vi "input_channel_task.vi"(8 "error in":errorcluster, 10 "Analog Input Channels":T2[](array[typedef])=[{"Channel Name"="Vapor Mass Flow", "Physical Channel"="cDAQ1Mod2/ai5", "Sensor Type"=enum."Mass Flow Rate", "Signal Type"=enum."Current", "Terminal Configuration"=-1, "Minimum Value"=0.004, "Maximum Value"=0.02, "TC Type"=10086, "Sensor Min"=0.0, "Sensor Max"=50.0, "Sensor Offset"=0.0, "Sensor Unit"=enum."g/s", "Output Unit"=enum."g/s", "Unit Conversion"=1.0, "Active"=TRUE}, {"Channel Name"="Vapor Line Density", "Physical Channel"="cDAQ1Mod2/ai6", "Sensor Type"=enum."Density", "Signal Type"=enum."Current", "Terminal Configuration"=-1, "Minimum Value"=0.004, "Maximum Value"=0.02, "TC Type"=10086, "Sensor Min"=0.0, "Sensor Max"=50.0, "Sensor Offset"=0.0, "Sensor Unit"=enum."g/cm3", "Output Unit"=enum."g/cm3", "Unit Conversion"=1.0, "Active"=TRUE}, {"Channel Name"="Liquid Mass Flow", "Physical Channel"="cDAQ1Mod2/ai3", "Sensor Type"=enum."Mass Flow Rate", "Signal Type"=enum."Current", "Terminal Configuration"=-1, "Minimum Value"=0.004, "Maximum Value"=0.02, "TC Type"=10086, "Sensor Min"=0.0, "Sensor Max"=50.0, "Sensor Offset"=0.0, "Sensor Unit"=enum."g/s", "Output Unit"=enum."g/s", "Unit Conversion"=1.0, "Active"=TRUE}, {"Channel Name"="Liquid Line Density", "Physical Channel"="cDAQ1Mod2/ai4", "Sensor Type"=enum."Density", "Signal Type"=enum."Current", "Terminal Configuration"=-1, "Minimum Value"=0.004, "Maximum Value"=0.02, "TC Type"=10086, "Sensor Min"=0.0, "Sensor Max"=50.0, "Sensor Offset"=0.0, "Sensor Unit"=enum."g/cm3", "Output Unit"=enum."g/cm3", "Unit Conversion"=1.0, "Active"=TRUE}, {"Channel Name"="Vapor Tank Pressure", "Physical Channel"="cDAQ1Mod5/ai1", "Sensor Type"=enum."Absolute Pressure", "Signal Type"=enum."Voltage", "Terminal Configuration"=-1, "Minimum Value"=0.0, "Maximum Value"=5.0, "TC Type"=10086, "Sensor Min"=0.0, "Sensor Max"=50.0, "Sensor Offset"=0.0, "Sensor Unit"=enum."psi", "Output Unit"=enum."Pa", "Unit Conversion"=6894.75729, "Active"=TRUE}, {"Channel Name"="Liquid Tank Pressure", "Physical Channel"="cDAQ1Mod5/ai2", "Sensor Type"=enum."Absolute Pressure", "Signal Type"=enum."Voltage", "Terminal Configuration"=-1, "Minimum Value"=0.0, "Maximum Value"=5.0, "TC Type"=10086, "Sensor Min"=0.0, "Sensor Max"=50.0, "Sensor Offset"=0.0, "Sensor Unit"=enum."psi", "Output Unit"=enum."Pa", "Unit Conversion"=6894.75729, "Active"=TRUE}, {"Channel Name"="Separator Pressure", "Physical Channel"="cDAQ1Mod5/ai0", "Sensor Type"=enum."Absolute Pressure", "Signal Type"=enum."Voltage", "Terminal Configuration"=-1, "Minimum Value"=0.0, "Maximum Value"=5.0, "TC Type"=10086, "Sensor Min"=0.0, "Sensor Max"=50.0, "Sensor Offset"=0.0, "Sensor Unit"=enum."psi", "Output Unit"=enum."Pa", "Unit Conversion"=6894.75729, "Active"=TRUE}, {"Channel Name"="Liquid Inlet Pressure", "Physical Channel"="cDAQ1Mod5/ai4", "Sensor Type"=enum."Absolute Pressure", "Signal Type"=enum."Voltage", "Terminal Configuration"=-1, "Minimum Value"=0.0, "Maximum Value"=5.0, "TC Type"=10086, "Sensor Min"=0.0, "Sensor Max"=50.0, "Sensor Offset"=0.0, "Sensor Unit"=enum."psi", "Output Unit"=enum."Pa", "Unit Conversion"=6894.75729, "Active"=TRUE}, {"Channel Name"="Vapor Inlet Pressure", "Physical Channel"="cDAQ1Mod5/ai3", "Sensor Type"=enum."Absolute Pressure", "Signal Type"=enum."Voltage", "Terminal Configuration"=-1, "Minimum Value"=0.0, "Maximum Value"=5.0, "TC Type"=10086, "Sensor Min"=0.0, "Sensor Max"=50.0, "Sensor Offset"=0.0, "Sensor Unit"=enum."psi", "Output Unit"=enum."Pa", "Unit Conversion"=6894.75729, "Active"=TRUE}, {"Channel Name"="Vapor Tank Temperature", "Physical Channel"="cDAQ1Mod6/ai1", "Sensor Type"=enum."Temperature", "Signal Type"=enum."Temperature", "Terminal Configuration"=-1, "Minimum Value"=0.0, "Maximum Value"=100.0, "TC Type"=10086, "Sensor Min"=0.0, "Sensor Max"=50.0, "Sensor Offset"=0.0, "Sensor Unit"=enum."C", "Output Unit"=enum."C", "Unit Conversion"=1.0, "Active"=TRUE}, {"Channel Name"="Vapor Inlet Temperature", "Physical Channel"="cDAQ1Mod7/ai2", "Sensor Type"=enum."Temperature", "Signal Type"=enum."Temperature", "Terminal Configuration"=-1, "Minimum Value"=0.0, "Maximum Value"=100.0, "TC Type"=10086, "Sensor Min"=0.0, "Sensor Max"=50.0, "Sensor Offset"=0.0, "Sensor Unit"=enum."C", "Output Unit"=enum."C", "Unit Conversion"=1.0, "Active"=TRUE}, {"Channel Name"="Liquid Tank Temperature", "Physical Channel"="cDAQ1Mod6/ai2", "Sensor Type"=enum."Temperature", "Signal Type"=enum."Temperature", "Terminal Configuration"=-1, "Minimum Value"=0.0, "Maximum Value"=100.0, "TC Type"=10086, "Sensor Min"=0.0, "Sensor Max"=50.0, "Sensor Offset"=0.0, "Sensor Unit"=enum."C", "Output Unit"=enum."C", "Unit Conversion"=1.0, "Active"=TRUE}, {"Channel Name"="Liquid Inlet Temperature", "Physical Channel"="cDAQ1Mod7/ai3", "Sensor Type"=enum."Temperature", "Signal Type"=enum."Temperature", "Terminal Configuration"=-1, "Minimum Value"=0.0, "Maximum Value"=100.0, "TC Type"=10086, "Sensor Min"=0.0, "Sensor Max"=50.0, "Sensor Offset"=0.0, "Sensor Unit"=enum."C", "Output Unit"=enum."C", "Unit Conversion"=1.0, "Active"=TRUE}, {"Channel Name"="Separator Temperature", "Physical Channel"="cDAQ1Mod6/ai0", "Sensor Type"=enum."Temperature", "Signal Type"=enum."Temperature", "Terminal Configuration"=-1, "Minimum Value"=0.0, "Maximum Value"=100.0, "TC Type"=10086, "Sensor Min"=0.0, "Sensor Max"=50.0, "Sensor Offset"=0.0, "Sensor Unit"=enum."C", "Output Unit"=enum."C", "Unit Conversion"=1.0, "Active"=TRUE}, {"Channel Name"="Lower Dev Section Pressure", "Physical Channel"="cDAQ1Mod5/ai6", "Sensor Type"=enum."Absolute Pressure", "Signal Type"=enum."Voltage", "Terminal Configuration"=-1, "Minimum Value"=0.0, "Maximum Value"=5.0, "TC Type"=10086, "Sensor Min"=0.0, "Sensor Max"=50.0, "Sensor Offset"=0.0, "Sensor Unit"=enum."psi", "Output Unit"=enum."Pa", "Unit Conversion"=6894.75729, "Active"=TRUE}, {"Channel Name"="Upper Dev Section Temperature", "Physical Channel"="cDAQ1Mod6/ai3", "Sensor Type"=enum."Temperature", "Signal Type"=enum."Temperature", "Terminal Configuration"=-1, "Minimum Value"=0.0, "Maximum Value"=100.0, "TC Type"=10086, "Sensor Min"=0.0, "Sensor Max"=50.0, "Sensor Offset"=0.0, "Sensor Unit"=enum."C", "Output Unit"=enum."C", "Unit Conversion"=1.0, "Active"=TRUE}, {"Channel Name"="Upper Dev Section Pressure", "Physical Channel"="cDAQ1Mod5/ai5", "Sensor Type"=enum."Absolute Pressure", "Signal Type"=enum."Voltage", "Terminal Configuration"=-1, "Minimum Value"=0.0, "Maximum Value"=5.0, "TC Type"=10086, "Sensor Min"=0.0, "Sensor Max"=50.0, "Sensor Offset"=0.0, "Sensor Unit"=enum."psi", "Output Unit"=enum."Pa", "Unit Conversion"=6894.75729, "Active"=TRUE}, {"Channel Name"="Test Section Temperature", "Physical Channel"="cDAQ1Mod6/ai10", "Sensor Type"=enum."Temperature", "Signal Type"=enum."Temperature", "Terminal Configuration"=-1, "Minimum Value"=0.0, "Maximum Value"=100.0, "TC Type"=10086, "Sensor Min"=0.0, "Sensor Max"=50.0, "Sensor Offset"=0.0, "Sensor Unit"=enum."C", "Output Unit"=enum."C", "Unit Conversion"=1.0, "Active"=TRUE}, {"Channel Name"="Mixing Tee dP", "Physical Channel"="cDAQ1Mod5/ai9", "Sensor Type"=enum."Differential Pressure", "Signal Type"=enum."Voltage", "Terminal Configuration"=-1, "Minimum Value"=0.05, "Maximum Value"=5.05, "TC Type"=10086, "Sensor Min"=0.0, "Sensor Max"=50.0, "Sensor Offset"=0.0, "Sensor Unit"=enum."psi", "Output Unit"=enum."Pa", "Unit Conversion"=6894.75729, "Active"=TRUE}, {"Channel Name"="PG inlet-Mixing Tee Pressure", "Physical Channel"="cDAQ1Mod5/ai10", "Sensor Type"=enum."Absolute Pressure", "Signal Type"=enum."Voltage", "Terminal Configuration"=-1, "Minimum Value"=0.0, "Maximum Value"=5.0, "TC Type"=10086, "Sensor Min"=0.0, "Sensor Max"=50.0, "Sensor Offset"=0.0, "Sensor Unit"=enum."psi", "Output Unit"=enum."Pa", "Unit Conversion"=6894.75729, "Active"=TRUE}, {"Channel Name"="PG inlet-Mixing Tee Temperature", "Physical Channel"="cDAQ1Mod7/ai6", "Sensor Type"=enum."Temperature", "Signal Type"=enum."Temperature", "Terminal Configuration"=-1, "Minimum Value"=0.0, "Maximum Value"=100.0, "TC Type"=10073, "Sensor Min"=0.0, "Sensor Max"=50.0, "Sensor Offset"=0.0, "Sensor Unit"=enum."C", "Output Unit"=enum."C", "Unit Conversion"=1.0, "Active"=TRUE}, {"Channel Name"="Atmospheric Pressure", "Physical Channel"="cDAQ1Mod5/ai8", "Sensor Type"=enum."Absolute Pressure", "Signal Type"=enum."Voltage", "Terminal Configuration"=-1, "Minimum Value"=1.0, "Maximum Value"=5.0, "TC Type"=10086, "Sensor Min"=0.0, "Sensor Max"=50.0, "Sensor Offset"=0.0, "Sensor Unit"=enum."psi", "Output Unit"=enum."Pa", "Unit Conversion"=6894.75729, "Active"=TRUE}, {"Channel Name"="PG Absolute Pressure", "Physical Channel"="cDAQ1Mod5/ai11", "Sensor Type"=enum."Absolute Pressure", "Signal Type"=enum."Voltage", "Terminal Configuration"=-1, "Minimum Value"=0.0, "Maximum Value"=5.0, "TC Type"=10086, "Sensor Min"=0.0, "Sensor Max"=50.0, "Sensor Offset"=0.0, "Sensor Unit"=enum."psi", "Output Unit"=enum."Pa", "Unit Conversion"=6894.75729, "Active"=TRUE}, {"Channel Name"="PG Pitot dP", "Physical Channel"="cDAQ1Mod2/ai7", "Sensor Type"=enum."Differential Pressure", "Signal Type"=enum."Current", "Terminal Configuration"=-1, "Minimum Value"=0.004, "Maximum Value"=0.02, "TC Type"=10086, "Sensor Min"=0.0, "Sensor Max"=50.0, "Sensor Offset"=0.0, "Sensor Unit"=enum."psi", "Output Unit"=enum."Pa", "Unit Conversion"=6894.75729, "Active"=TRUE}, {"Channel Name"="Vapor Line Pitot dP", "Physical Channel"="", "Sensor Type"=enum."Differential Pressure", "Signal Type"=enum."Current", "Terminal Configuration"=-1, "Minimum Value"=0.004, "Maximum Value"=0.02, "TC Type"=10086, "Sensor Min"=0.0, "Sensor Max"=50.0, "Sensor Offset"=0.0, "Sensor Unit"=enum."psi", "Output Unit"=enum."Pa", "Unit Conversion"=6894.75729, "Active"=FALSE}, {"Channel Name"="PG Vapor Temperature", "Physical Channel"="cDAQ1Mod7/ai4", "Sensor Type"=enum."Temperature", "Signal Type"=enum."Temperature", "Terminal Configuration"=-1, "Minimum Value"=0.0, "Maximum Value"=100.0, "TC Type"=10073, "Sensor Min"=0.0, "Sensor Max"=50.0, "Sensor Offset"=0.0, "Sensor Unit"=enum."C", "Output Unit"=enum."C", "Unit Conversion"=1.0, "Active"=TRUE}, {"Channel Name"="PG Liquid Temperature", "Physical Channel"="cDAQ1Mod7/ai5", "Sensor Type"=enum."Temperature", "Signal Type"=enum."Temperature", "Terminal Configuration"=-1, "Minimum Value"=0.0, "Maximum Value"=100.0, "TC Type"=10073, "Sensor Min"=0.0, "Sensor Max"=50.0, "Sensor Offset"=0.0, "Sensor Unit"=enum."C", "Output Unit"=enum."C", "Unit Conversion"=1.0, "Active"=TRUE}, {"Channel Name"=" Window 1 to 4 dP", "Physical Channel"="cDAQ1Mod2/ai2", "Sensor Type"=enum."Differential Pressure", "Signal Type"=enum."Current", "Terminal Configuration"=-1, "Minimum Value"=0.004, "Maximum Value"=0.02, "TC Type"=10086, "Sensor Min"=0.0, "Sensor Max"=50.0, "Sensor Offset"=0.0, "Sensor Unit"=enum."inH2O", "Output Unit"=enum."Pa", "Unit Conversion"=248.84, "Active"=TRUE}, {"Channel Name"="Window 1 to 7 dP", "Physical Channel"="cDAQ1Mod2/ai1", "Sensor Type"=enum."Differential Pressure", "Signal Type"=enum."Current", "Terminal Configuration"=-1, "Minimum Value"=0.004, "Maximum Value"=0.02, "TC Type"=10086, "Sensor Min"=0.0, "Sensor Max"=50.0, "Sensor Offset"=0.0, "Sensor Unit"=enum."inH2O", "Output Unit"=enum."Pa", "Unit Conversion"=248.84, "Active"=TRUE}, {"Channel Name"="Window 1 to 7 Fast dP", "Physical Channel"="cDAQ1Mod2/ai0", "Sensor Type"=enum."Differential Pressure", "Signal Type"=enum."Current", "Terminal Configuration"=-1, "Minimum Value"=0.004, "Maximum Value"=0.02, "TC Type"=10086, "Sensor Min"=0.0, "Sensor Max"=50.0, "Sensor Offset"=0.0, "Sensor Unit"=enum."psi", "Output Unit"=enum."Pa", "Unit Conversion"=6894.75729, "Active"=TRUE}, {"Channel Name"="Camera Voltage", "Physical Channel"="cDAQ1Mod8/ai0", "Sensor Type"=enum."Other", "Signal Type"=enum."Voltage", "Terminal Configuration"=-1, "Minimum Value"=0.0, "Maximum Value"=10.0, "TC Type"=10086, "Sensor Min"=0.0, "Sensor Max"=50.0, "Sensor Offset"=0.0, "Sensor Unit"=enum."Volt", "Output Unit"=enum."Volt", "Unit Conversion"=1.0, "Active"=TRUE}, {"Channel Name"="TS Window 1 Temperature", "Physical Channel"="cDAQ1Mod6/ai4", "Sensor Type"=enum."Temperature", "Signal Type"=enum."Temperature", "Terminal Configuration"=-1, "Minimum Value"=0.0, "Maximum Value"=100.0, "TC Type"=10073, "Sensor Min"=0.0, "Sensor Max"=50.0, "Sensor Offset"=0.0, "Sensor Unit"=enum."C", "Output Unit"=enum."C", "Unit Conversion"=1.0, "Active"=TRUE}, {"Channel Name"="TS Window 7 Temperature", "Physical Channel"="cDAQ1Mod6/ai5", "Sensor Type"=enum."Temperature", "Signal Type"=enum."Temperature", "Terminal Configuration"=-1, "Minimum Value"=0.0, "Maximum Value"=100.0, "TC Type"=10073, "Sensor Min"=0.0, "Sensor Max"=50.0, "Sensor Offset"=0.0, "Sensor Unit"=enum."C", "Output Unit"=enum."C", "Unit Conversion"=1.0, "Active"=TRUE}, {"Channel Name"="TS Window 1 Absolute Pressure", "Physical Channel"="cDAQ1Mod5/ai12", "Sensor Type"=enum."Absolute Pressure", "Signal Type"=enum."Voltage", "Terminal Configuration"=-1, "Minimum Value"=0.0, "Maximum Value"=5.0, "TC Type"=10086, "Sensor Min"=0.0, "Sensor Max"=50.0, "Sensor Offset"=0.0, "Sensor Unit"=enum."psi", "Output Unit"=enum."Pa", "Unit Conversion"=6894.75729, "Active"=TRUE}, {"Channel Name"="TS Window 7 Absolute Pressure", "Physical Channel"="cDAQ1Mod5/ai13", "Sensor Type"=enum."Absolute Pressure", "Signal Type"=enum."Voltage", "Terminal Configuration"=-1, "Minimum Value"=0.0, "Maximum Value"=5.0, "TC Type"=10086, "Sensor Min"=0.0, "Sensor Max"=50.0, "Sensor Offset"=0.0, "Sensor Unit"=enum."psi", "Output Unit"=enum."Pa", "Unit Conversion"=6894.75729, "Active"=TRUE}, {"Channel Name"="Main Diode", "Physical Channel"="cDAQ1Mod8/ai1", "Sensor Type"=enum."Other", "Signal Type"=enum."Voltage", "Terminal Configuration"=-1, "Minimum Value"=0.0, "Maximum Value"=10.0, "TC Type"=10086, "Sensor Min"=0.0, "Sensor Max"=50.0, "Sensor Offset"=0.0, "Sensor Unit"=enum."Volt", "Output Unit"=enum."Volt", "Unit Conversion"=1.0, "Active"=TRUE}, {"Channel Name"="Control Diode", "Physical Channel"="cDAQ1Mod8/ai2", "Sensor Type"=enum."Other", "Signal Type"=enum."Voltage", "Terminal Configuration"=-1, "Minimum Value"=0.0, "Maximum Value"=10.0, "TC Type"=10086, "Sensor Min"=0.0, "Sensor Max"=50.0, "Sensor Offset"=0.0, "Sensor Unit"=enum."Volt", "Output Unit"=enum."Volt", "Unit Conversion"=1.0, "Active"=TRUE}, {"Channel Name"="TS Exterior Temperature", "Physical Channel"="cDAQ1Mod6/ai6", "Sensor Type"=enum."Temperature", "Signal Type"=enum."Temperature", "Terminal Configuration"=-1, "Minimum Value"=0.0, "Maximum Value"=100.0, "TC Type"=10073, "Sensor Min"=0.0, "Sensor Max"=50.0, "Sensor Offset"=0.0, "Sensor Unit"=enum."C", "Output Unit"=enum."C", "Unit Conversion"=1.0, "Active"=TRUE}, {"Channel Name"="DS Exterior Temperature", "Physical Channel"="cDAQ1Mod6/ai7", "Sensor Type"=enum."Temperature", "Signal Type"=enum."Temperature", "Terminal Configuration"=-1, "Minimum Value"=0.0, "Maximum Value"=100.0, "TC Type"=10073, "Sensor Min"=0.0, "Sensor Max"=50.0, "Sensor Offset"=0.0, "Sensor Unit"=enum."C", "Output Unit"=enum."C", "Unit Conversion"=1.0, "Active"=TRUE}] {"Unit Conversion" format="%0.5f"; "TC Type" items=["J"=10072, "K"=10073, "N"=10077, "R"=10082, "S"=10085, "T"=10086, "B"=10047, "E"=10055]; "Sensor Offset" format="%0.5f"; "Sensor Max" format="%0.5f"; "Sensor Min" format="%0.5f"; "Maximum Value" format="%0.5f"; "Minimum Value" format="%0.5f"; "Terminal Configuration" items=["Default"=-1, "RSE"=10083, "NRSE"=10078, "Differential"=10106, "Pseudodifferential"=12529]}) -> (0 "error out":errorcluster, 2 "Active Analog Channel-Data Packages":T1[](array[typedef]) {"Analog Input Channel"."Unit Conversion" format="%0.5f"; "Analog Input Channel"."TC Type" items=["J"=10072, "K"=10073, "N"=10077, "R"=10082, "S"=10085, "T"=10086, "B"=10047, "E"=10055]; "Analog Input Channel"."Sensor Offset" format="%0.5f"; "Analog Input Channel"."Sensor Max" format="%0.5f"; "Analog Input Channel"."Sensor Min" format="%0.5f"; "Analog Input Channel"."Maximum Value" format="%0.5f"; "Analog Input Channel"."Minimum Value" format="%0.5f"; "Analog Input Channel"."Terminal Configuration" items=["Default"=-1, "RSE"=10083, "NRSE"=10078, "Differential"=10106, "Pseudodifferential"=12529]}, 3 "task out":refnum<k21>)   [LabVIEW 2017]
uses:
  input_channel.ctl
  Box/Annular Flow/Jason/LabVIEW 2017/Input Channel Lists/analog_data_channel_pkg.ctl
  Box/Annular Flow/Jason/LabVIEW 2017/Input Channel Lists/analog_data.ctl
  <vilib>/DAQmx/create/channels.llb/DAQmx Create Channel (AI-Current-Basic).vi
  <vilib>/DAQmx/create/channels.llb/DAQmx Create Channel (AI-Voltage-Basic).vi
  <vilib>/DAQmx/create/channels.llb/DAQmx Create Channel (AI-Temperature-Thermocouple).vi
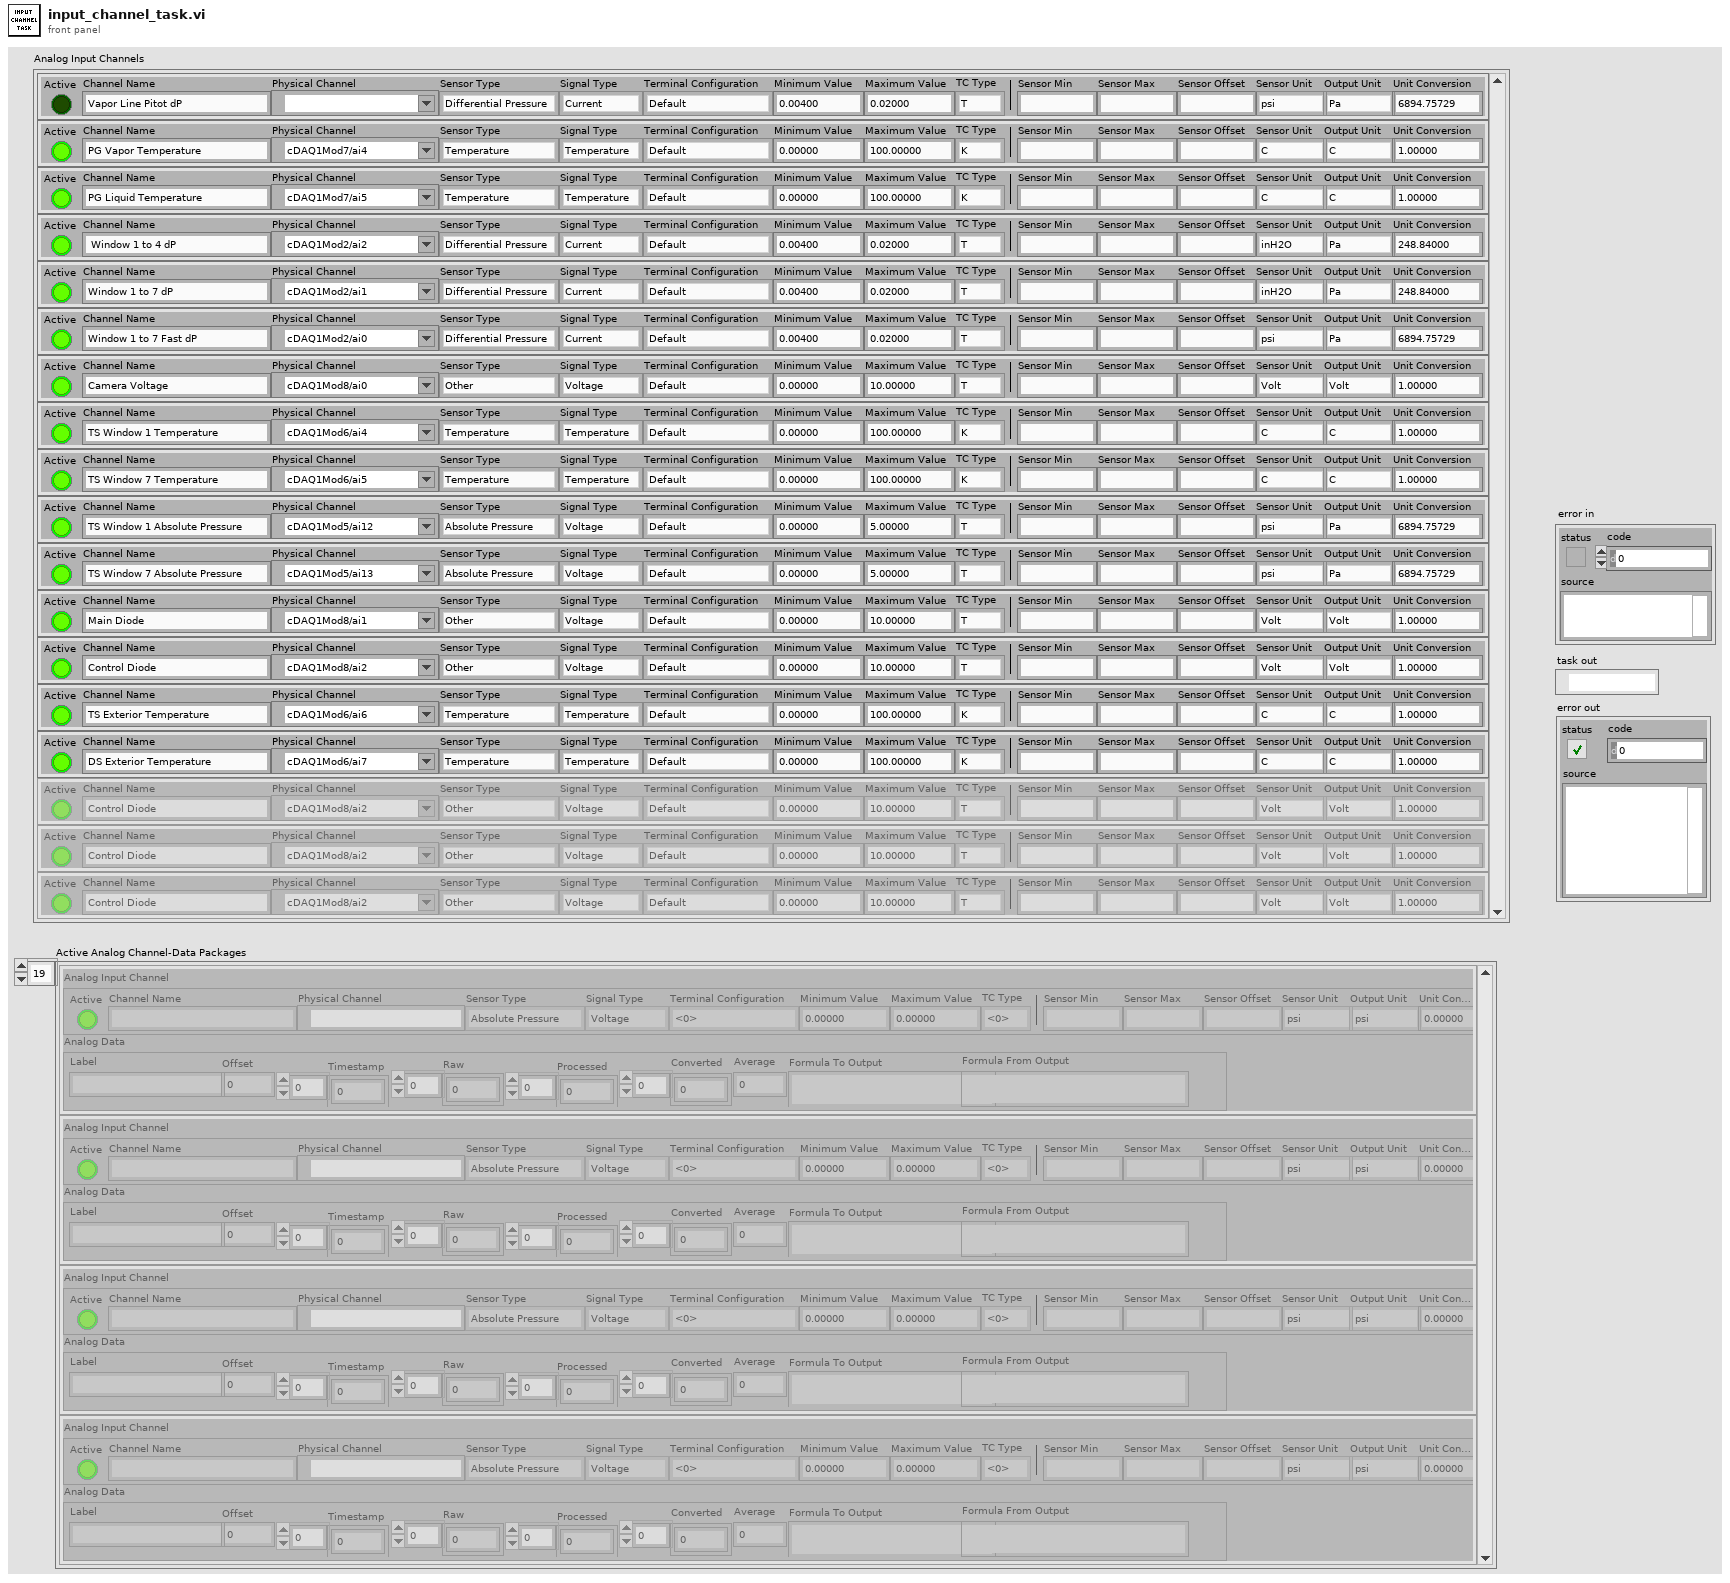
[diagram p1: front panel]
types:
  T1 = typedef "analog_data_channel_pkg.ctl" = cluster{"Analog Input Channel":T2, "Analog Data":T3}
  T2 = typedef "input_channel.ctl" = cluster{"Channel Name":string, "Physical Channel":tag, "Sensor Type":enum16{"Absolute Pressure", "Gauge Pressure", "Differential Pressure", "Temperature", "Mass Flow Rate", "Density", "Other"}, "Signal Type":enum16{"Voltage", "Current", "Temperature"}, "Terminal Configuration":i32, "Minimum Value":dbl, "Maximum Value":dbl, "TC Type":i32, "Sensor Min":dbl, "Sensor Max":dbl, "Sensor Offset":dbl, "Sensor Unit":enum16{"psi", "Pa", "inH2O", "inHg", "C", "K", "g/s", "g/cm3", "Volt", "Amp", ""}, "Output Unit":enum16{"psi", "Pa", "inH2O", "inHg", "C", "K", "g/s", "g/cm3", "Volt", "Amp", ""}, "Unit Conversion":dbl, "Active":bool}
  T3 = typedef "analog_data.ctl" = cluster{"Label":string, "Offset":dbl, "Timestamp":dbl[], "Raw":dbl[], "Processed":dbl[], "Converted":dbl[], "Average":dbl, "Formula To Output":string, "Formula From Output":string}
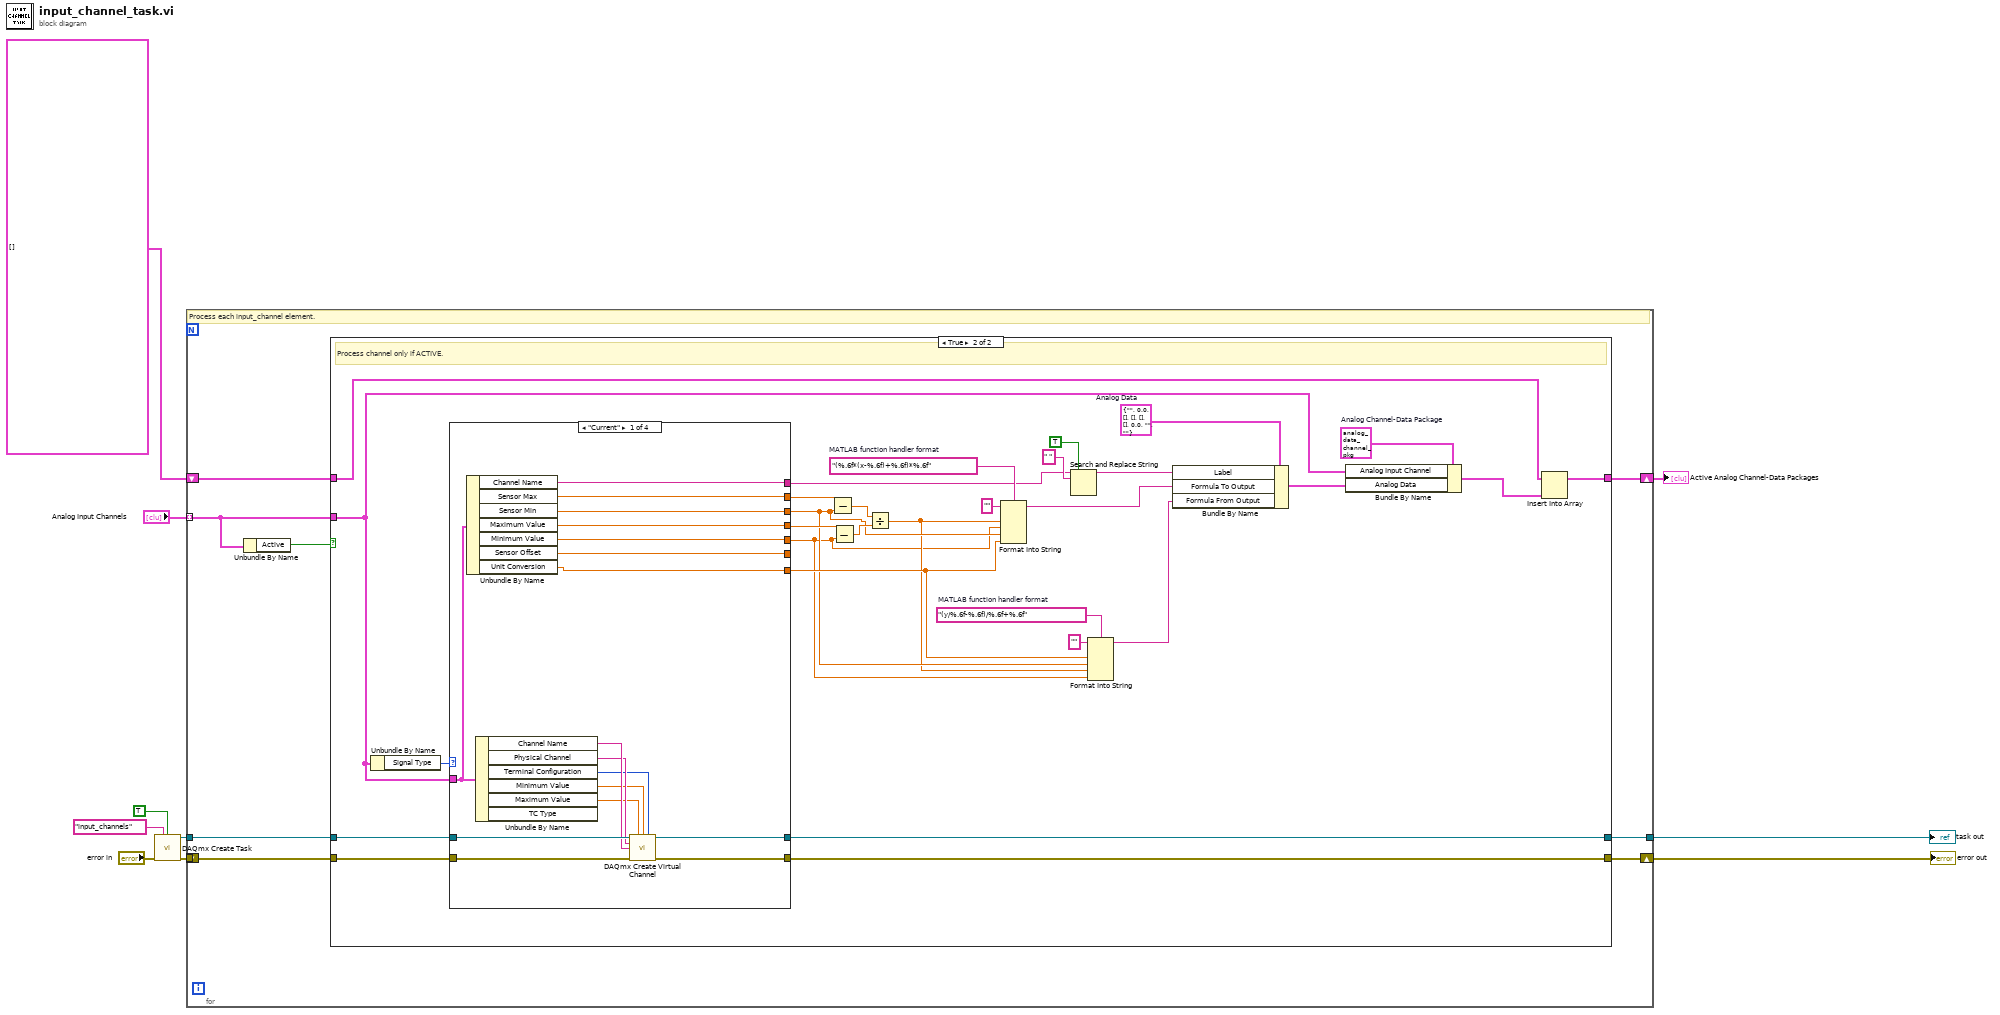
[diagram p0: block diagram]
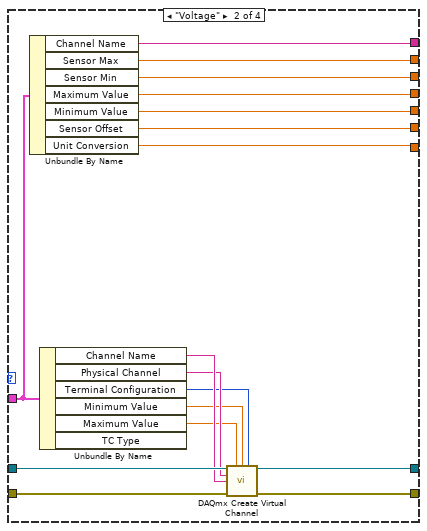
[diagram p3: hidden frame]
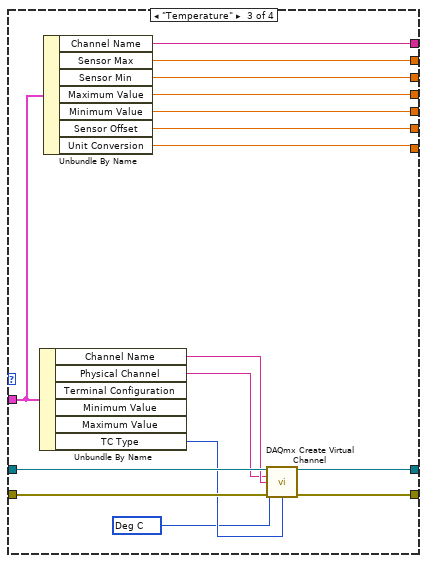
[diagram p4: hidden frame]
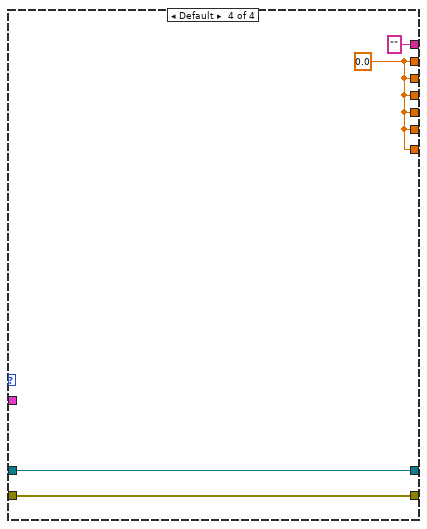
[diagram p5: hidden frame]
diagram:
  n1 = call <vilib>:"DAQmx Create Task.vi"("new task name"="input_channels", "auto cleanup"=TRUE, "error in"="error in") -> ("task out"=w7:refnum<k21>, "error out"=w6:errorcluster)  [unwired: 11 in]
  n2 = for {
    tunnel: "Analog Input Channels" -> [w13] mode=indexing
    tunnel: w7 -> [w18]
    tunnel: w6 -> [w17]
    tunnel: [w16] -> w4
    shift-right: [w14] -> w1
    shift-left: T1[] [] ("Array") -> [w11]
    shift-right: [w15] -> w3
    shift-left: _ -> [_]
    # "Process each input_channel element."
    n3 = Unbundle By Name(w13) -> ("Active"=w12:bool)
    n4 = case shown="True" w12 {
      tunnel: w18 -> [w21 w50]
      tunnel: w17 -> [w20 w49]
      tunnel: [w21 w48] -> w16
      tunnel: [w20 w22] -> w15
      tunnel: w13 -> [_ w27]
      tunnel: [w19 w24] -> w14
      tunnel: w11 -> [w19 w25]
      frame False {
        # "Skip Channel if NOT ACTIVE."
      }
      frame True {
        w29 = T1 {"Analog Input Channel"={"Channel Name"="", "Physical Channel"="", "Sensor Type"=enum."Absolute Pressure", "Signal Type"=enum."Voltage", "Terminal Configuration"=-1, "Minimum Value"=5.0, "Maximum Value"=5.0, "TC Type"=10072, "Sensor Min"=5.0, "Sensor Max"=5.0, "Sensor Offset"=5.0, "Sensor Unit"=enum."psi", "Output Unit"=enum."psi", "Unit Conversion"=5.0, "Active"=TRUE}, "Analog Data"={"Label"="", "Offset"=0.0, "Timestamp"=[], "Raw"=[], "Processed"=[], "Converted"=[], "Average"=0.0, "Formula To Output"="", "Formula From Output"=""}}  # Analog Channel-Data Package
        w36 = "(y/%.6f-%.6f)/%.6f+%.6f"  # MATLAB function handler format
        w47 = T3 {"Label"="", "Offset"=0.0, "Timestamp"=[], "Raw"=[], "Processed"=[], "Converted"=[], "Average"=0.0, "Formula To Output"="", "Formula From Output"=""}  # Analog Data
        w39 = "(%.6f*(x-%.6f)+%.6f)*%.6f"  # MATLAB function handler format
        # "Process channel only if ACTIVE."
        n5 = Unbundle By Name(w27) -> ("Signal Type"=w51:enum16{"Voltage", "Current", "Temperature"})
        n6 = case shown="\"Current\"" w51 {
          tunnel: w50 -> [w68 w85 w99 w105]
          tunnel: w49 -> [w67 w82 w98 w104]
          tunnel: [w63 w84 w101 w105] -> w48
          tunnel: [w62 w83 w100 w104] -> w22
          tunnel: w27 -> [w55 w70 w94 _]
          tunnel: [w61 w76 w93 "" ("Channel Name")] -> w26
          tunnel: [w60 w75 w92 w102] -> w43
          tunnel: [w59 w74 w91 w102] -> w32
          tunnel: [w58 w73 w90 w102] -> w42
          tunnel: [w57 w72 w89 w102] -> w30
          tunnel: [w56 w71 w88 w102] -> _
          tunnel: [w54 w69 w87 w102] -> w33
          frame "Current" {
            n7 = Unbundle By Name(w55) -> ("Channel Name"=w61:string, "Sensor Max"=w60:dbl, "Sensor Min"=w59:dbl, "Maximum Value"=w58:dbl, "Minimum Value"=w57:dbl, "Sensor Offset"=w56:dbl, "Unit Conversion"=w54:dbl)
            n8 = Unbundle By Name(w55) -> ("Channel Name"=w66:string, "Physical Channel"=w65:tag, "Terminal Configuration"=w64:i32, "Minimum Value"=w53:dbl, "Maximum Value"=w52:dbl)  [unwired: 1 out]
            n9 = call-poly <vilib>:"DAQmx Create Virtual Channel.vi"("task in"=w68, "maximum value"=w52, "minimum value"=w53, "input terminal configuration"=w64, "physical channels"=w65, "name to assign"=w66, "error in"=w67) -> ("task out"=w63:refnum<k21>, "error out"=w62:errorcluster)  [unwired: 7 in]
          }
          frame "Voltage" {
            n10 = Unbundle By Name(w70) -> ("Channel Name"=w76:string, "Sensor Max"=w75:dbl, "Sensor Min"=w74:dbl, "Maximum Value"=w73:dbl, "Minimum Value"=w72:dbl, "Sensor Offset"=w71:dbl, "Unit Conversion"=w69:dbl)
            n11 = Unbundle By Name(w70) -> ("Channel Name"=w81:string, "Physical Channel"=w80:tag, "Terminal Configuration"=w77:i32, "Minimum Value"=w79:dbl, "Maximum Value"=w78:dbl)  [unwired: 1 out]
            n12 = call-poly <vilib>:"DAQmx Create Virtual Channel.vi"("task in"=w85, "maximum value"=w78, "minimum value"=w79, "input terminal configuration"=w77, "physical channels"=w80, "name to assign"=w81, "error in"=w82) -> ("task out"=w84:refnum<k21>, "error out"=w83:errorcluster)  [unwired: 7 in]
          }
          frame "Temperature" {
            w86 = 10143 items=["Deg C"=10143, "Deg F"=10144, "Kelvins"=10325, "Deg R"=10145, "From Custom Scale"=10065] ("units")
            n13 = Unbundle By Name(w94) -> ("Channel Name"=w96:string, "Physical Channel"=w95:tag, "TC Type"=w97:i32)  [unwired: 3 out]
            n14 = Unbundle By Name(w94) -> ("Channel Name"=w93:string, "Sensor Max"=w92:dbl, "Sensor Min"=w91:dbl, "Maximum Value"=w90:dbl, "Minimum Value"=w89:dbl, "Sensor Offset"=w88:dbl, "Unit Conversion"=w87:dbl)
            n15 = call-poly <vilib>:"DAQmx Create Virtual Channel.vi"("task in"=w99, "physical channels"=w95, "name to assign"=w96, "units"=w86, "error in"=w98, "thermocouple type"=w97) -> ("task out"=w101:refnum<k21>, "error out"=w100:errorcluster)  [unwired: 8 in]
          }
          frame Default {
            w102 = 0.0
          }
        }
        n16 = Subtract(x=w43, y=w32) -> (x-y=w40:dbl)
        n17 = Subtract(x=w42, y=w30) -> (x-y=w41:dbl)
        n18 = Divide(x=w40, y=w41) -> (x/y=w31:dbl)
        n19 = Format Into String(format string=w39, initial string="", w31, w30, w32, w33) -> (resulting string=w37:string)  [unwired: 1 in, 1 out]
        n20 = Search and Replace String(replace all?=TRUE ("replace all? (F)"), input string=w26, search string=" ") -> (result string=w44:string)  [unwired: 5 in, 3 out]
        n21 = Format Into String(format string=w36, initial string="", w33, w32, w31, w30) -> (resulting string=w34:string)  [unwired: 1 in, 1 out]
        n22 = Bundle By Name(cluster=w47, "Label"=w44, "Formula To Output"=w37, "Formula From Output"=w34) -> (w28:T3)
        n23 = Bundle By Name(cluster=w29, "Analog Input Channel"=w27, "Analog Data"=w28) -> (w23:T1)
        n24 = Insert Into Array(array=w25, new element=w23) -> (w24:T1[])  [unwired: 1 in]
      }
    }
  }
  "Active Analog Channel-Data Packages" <- w1
  "task out" <- w4
  "error out" <- w3
